vi "Write FP Control Ref.vi"(8 "error in (no error)":errorcluster, 10 "FP Control Ref":T1, 11 "Main in":refnum<class "Main.lvclass">) -> (0 "error out":errorcluster, 3 "Main out":refnum<class "Main.lvclass">)   [LabVIEW 2023, in "GUI.lvlib" / "Main.lvlib" / "Main.lvclass"]
uses:
  Main.lvclass
  Typdefs/Main.App.Cluster.ctl
  Main.lvclass/Main.ctl
  GUI.lvlib
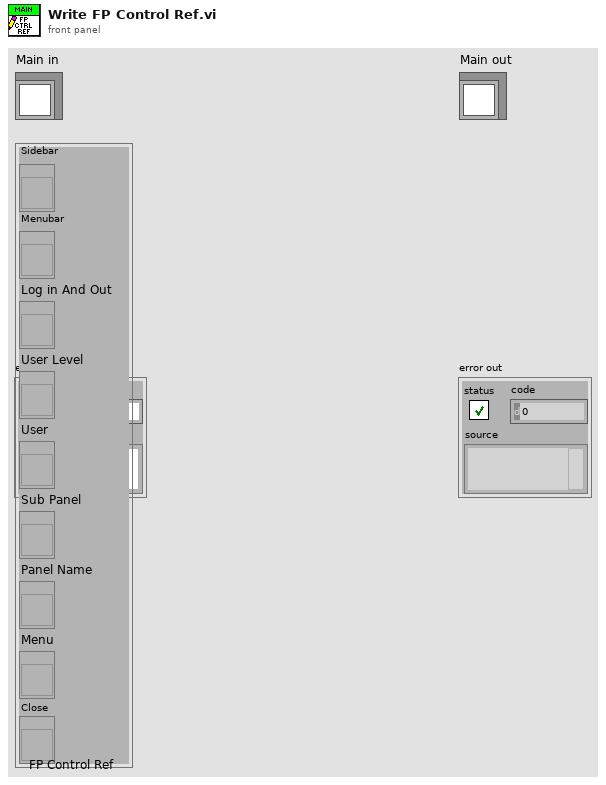
[diagram p1: front panel]
types:
  T1 = typedef "GUI.lvlib/Main.App.Cluster.ctl" = cluster{"Sidebar":refnum<vi>, "Menubar":refnum<vi>, "Log in And Out":refnum<vi>, "User Level":refnum<vi>, "User":refnum<vi>, "Sub Panel":refnum<vi>, "Panel Name":refnum<vi>, "Menu":refnum<vi>, "Close":refnum<vi>}
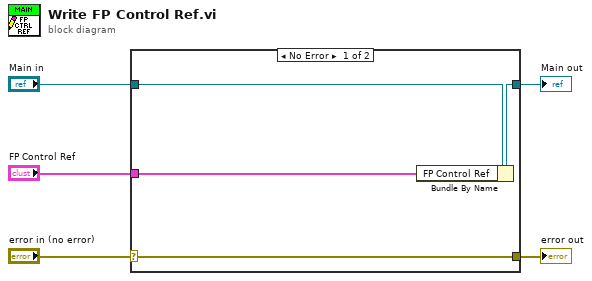
[diagram p0: block diagram]
diagram:
  n1 = case shown="No Error" "error in (no error)" {
    selector: "error in (no error)" -> [w9 w10]
    tunnel: [w9 w10] -> w4
    tunnel: [w7 w11] -> w2
    tunnel: "Main in" -> [w8 w11]
    tunnel: "FP Control Ref" -> [w6 _]
    frame No Error {
      n2 = Bundle By Name(cluster=w8, "FP Control Ref"=w6) -> (w7:refnum<class "Main.lvclass">)
    }
    frame Error {
    }
  }
  "error out" <- w4
  "Main out" <- w2
